vi "PH_DeformableMirror.evt call SetHV.vi"(0 "i ref in":refnum<vi>, 1 "Object":string="N/A", 3 "HV on/off":bool, 5 "error in (no error)":errorcluster) -> (14 "i ref out":refnum<vi>, 19 "error out":errorcluster)   [LabVIEW 2014, in "PH_DeformableMirror.lvlib"]
uses:
  PH_DeformableMirror.lvlib
  CSCore/CSSystem/CoreLib/CoreLib.short 2 byte array.vi
  CSCore/CSSystem/CoreLib/CoreLib.lvlib
  CSCore/BaseProcess/BaseProcess.lvlib
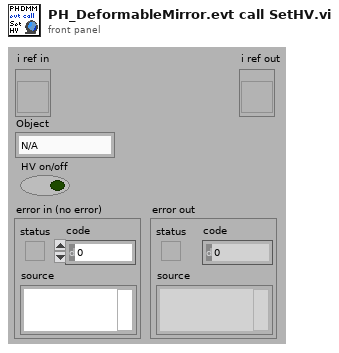
[diagram p1: front panel]
types:
  T1 = typedef "CoreDefs.rawDataType.ctl" = i8[]
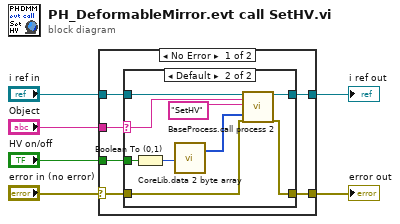
[diagram p0: block diagram]
diagram:
  n1 = case shown="No Error" "error in (no error)" {
    selector: "error in (no error)" -> [w9 w24]
    tunnel: "i ref in" -> [w12 w25]
    tunnel: [w11 w25] -> w5
    tunnel: [w10 w24] -> w4
    tunnel: "Object" -> [w8 _]
    tunnel: "HV on/off" -> [w7 _]
    frame No Error {
      n2 = case shown="Default" w8 {
        selector: w8 -> [_ w19]
        tunnel: w12 -> [w14 w23]
        tunnel: [w14 w22] -> w11
        tunnel: [w13 w21] -> w10
        tunnel: w9 -> [w13 w20]
        tunnel: w7 -> [_ w17]
        frame "N/A" {
        }
        frame Default {
          n3 = Boolean To (0,1)(Boolean=w17) -> (0, 1=w16:i16)
          n4 = call-poly "CoreLib.data 2 byte array.vi"("i16"=w16) -> ("byteArray out"=w15:T1)  [unwired: 18 in]
          n5 = call "BaseProcess.call process 2.vi"("i ref in"=w23, "Object"=w19, "Selector"="SetHV", "Data"=w15, "error in (no error)"=w20) -> ("i ref out"=w22:refnum<vi>, "error out"=w21:errorcluster)  [unwired: 13 in]
        }
      }
    }
    frame Error {
    }
  }
  "error out" <- w4
  "i ref out" <- w5
